vi "Process Pulse.vi"(8 "error in (no error)":errorcluster, 10 "Input":T2={"From"="broadcaster", "To"="broadcaster", "Pulse"=FALSE}, 11 "Module in":refnum<class "Module.lvclass">) -> (0 "error out":errorcluster, 2 "Outputs":T1(array[cluster]), 3 "Module out":refnum<class "Module.lvclass">)   [LabVIEW 2021, in "Module.lvclass"]
uses:
  Module.lvclass
  Module.lvclass/Module.ctl
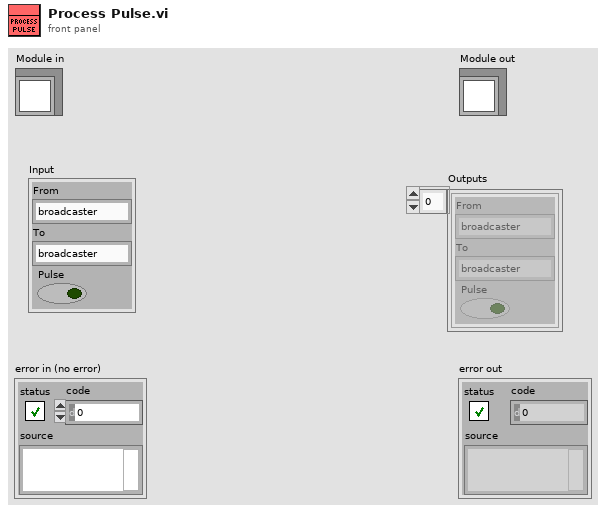
[diagram p1: front panel]
types:
  T1 = cluster{"From":string, "To":string, "Pulse":bool}[]
  T2 = cluster{"From":string, "To":string, "Pulse":bool}
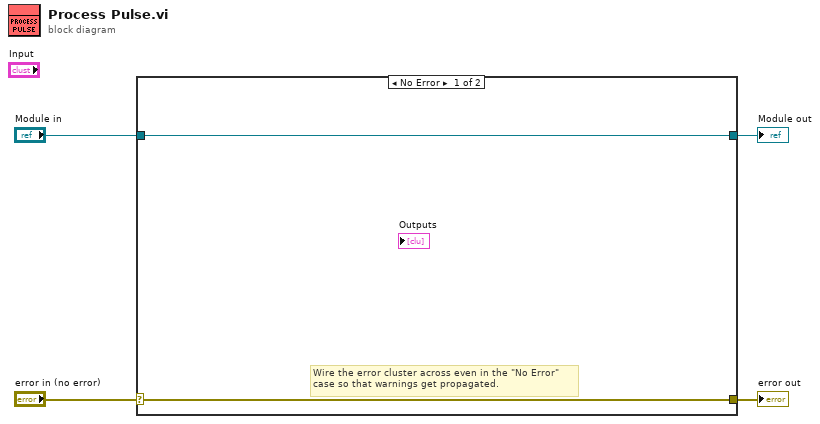
[diagram p0: block diagram]
diagram:
  n1 = case shown="No Error" "error in (no error)" {
    selector: "error in (no error)" -> [w5 w8]
    tunnel: [w5 w8] -> w3
    tunnel: [w6 w7] -> w1
    tunnel: "Module in" -> [w6 w7]
    frame No Error {
      # "Wire the error cluster across even in the \"No Error\"\ncase so that warnings get propagated."
    }
    frame Error {
    }
  }
  "error out" <- w3
  "Module out" <- w1
